vi "set RT data buffer.vi"(8 "error in (no error)":errorcluster) -> (0 "error out":errorcluster)   [LabVIEW 2024]
uses:
  cRIO VI parameters.vi
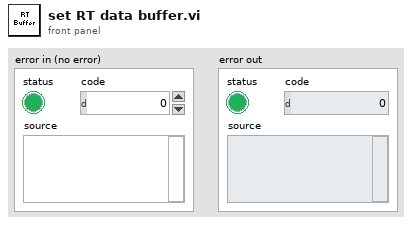
[diagram p1: front panel]
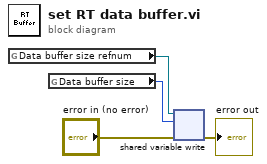
[diagram p0: block diagram]
diagram:
  n1 = global read "cRIO VI parameters.vi" "Data buffer size refnum"() -> (w2:refnum<k21>)
  n2 = global read "cRIO VI parameters.vi" "Data buffer size"() -> (w1:i32)
  n3 = shared-variable-write(w2, "error in (no error)", w1) -> (→"error out":errorcluster)  [unwired: 1 out]
